vi "Power_Supply Verify Instrument Options - Versions.vi"(8 "error in (no error)":errorcluster, 11 "N6702A in":refnum<class "N6700.lvclass">) -> (0 "error out":errorcluster, 3 "N6702A out":refnum<class "N6700.lvclass">)   [LabVIEW 2018, in "N6700.lvclass"]
uses:
  N6700.lvclass
  Controls/Instrument Attributes Cluster.ctl
  N6700.lvclass/N6700.ctl
  <instrlib>/Agilent N6700 Series/Agilent N6700 Series.lvlib
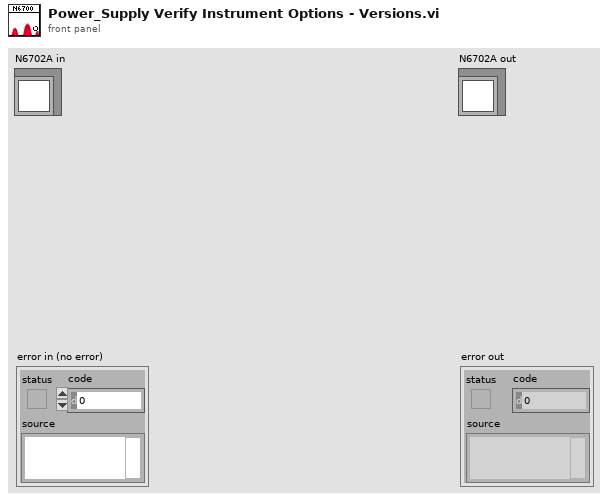
[diagram p1: front panel]
types:
  T1 = typedef "Instrument Attributes Cluster.ctl" = cluster{"Reported Firmware Rev":string, "Reported Options":string}
  T2 = typedef "Class Instrument Info.ctl" = string[]
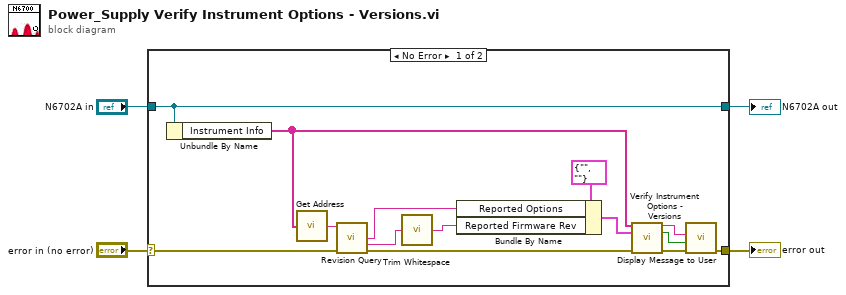
[diagram p0: block diagram]
diagram:
  n1 = case shown="No Error" "error in (no error)" {
    selector: "error in (no error)" -> [w8 w20]
    tunnel: [w15 w20] -> w3
    tunnel: [w14 w19] -> w1
    tunnel: "N6702A in" -> [w14 w19]
    frame No Error {
      n2 = Unbundle By Name(w14) -> ("Instrument Info"=w6:T2)
      n3 = call "Get Address.vi"("Instrument Info"=w6) -> ("Address"=w7:string)  [unwired: 4 in]
      n4 = call <instrlib>:"Revision Query.vi"("VISA resource name"=w7, "error in (no error)"=w8) -> ("Instrument Driver Revision"=w5:string, "Instrument Firmware Revision"=w9:string, "error out"=w10:errorcluster)  [unwired: 10 in, 1 out]
      n5 = call <vilib>:"Trim Whitespace.vi"("string"=w9) -> ("trimmed string"=w11:string)  [unwired: 1 in]
      n6 = Bundle By Name(cluster=T1 {"Reported Firmware Rev"="", "Reported Options"=""} ("Instrument Attributes"), "Reported Options"=w5, "Reported Firmware Rev"=w11) -> (w12:T1)
      n7 = call "Verify Instrument Options - Versions.vi"("Instrument Info"=w6, "Instrument Attributes"=w12, "error in (no error)"=w10) -> ("Options & Versions Validation"=w18:string, "Mismatch? (True = Mismatch)"=w17:bool, "error out"=w16:errorcluster)  [unwired: 10 in]
      n8 = call "Display Message to User"("error in (no error)"=w16, "Enable"=w17, "Message"=w18) -> ("error out"=w15:errorcluster)  [unwired: 7 in, 1 out]
    }
    frame Error {
    }
  }
  "N6702A out" <- w1
  "error out" <- w3
